vi "Sub_Read_Variable_Header.vi"(8 "error in (no error)":errorcluster, 9 "QoS":T1, 10 "Variable Header":u8[](array[numeric]) format="%x") -> (0 "error out":errorcluster, 1 "remaining bytes":u8[](array[numeric]) format="%x", 2 "Message ID":u16=1 format="%x", 3 "Topic Name":string="Topic")   [LabVIEW 2024, in "MQTT_Functions.lvlib"]
uses:
  MQTT_Functions.lvlib
  Controls/QoS.ctl
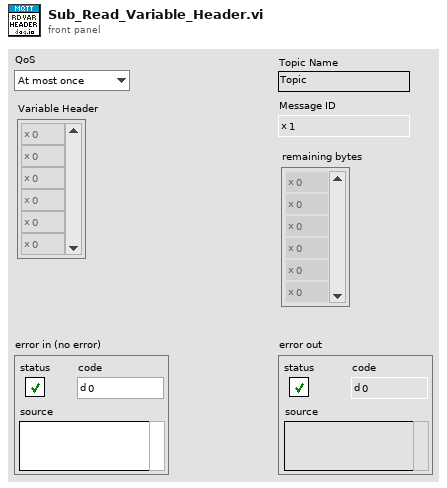
[diagram p1: front panel]
types:
  T1 = typedef "MQTT_Functions.lvlib/QoS.ctl" = enum8{"At most once", "At least once", "Exactly once", "Reserved"}
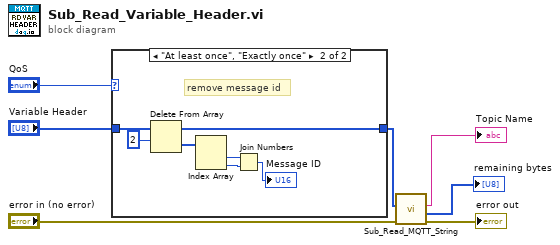
[diagram p0: block diagram]
diagram:
  n1 = case shown="\"At least once\", \"Exactly once\"" "QoS" {
    tunnel: "Variable Header" -> [w8 w15]
    tunnel: [w8 w9] -> w4
    frame "At most once", Default {
      # "no message id"
    }
    frame "At least once", "Exactly once" {
      # "remove message id"
      n2 = Delete From Array(array=w15, length=2) -> (deleted portion=w13:u8[], array with subset deleted=w9:u8[])  [unwired: 1 in]
      n3 = Index Array(array=w13) -> (element #1=w11:u8, element #2=w12:u8)  [unwired: 2 in]
      n4 = Join Numbers(hi=w11, lo=w12) -> ((hi.lo)=→"Message ID":u16)
    }
  }
  n5 = call "Sub_Read_MQTT_String.vi"("error in (no error)"="error in (no error)", "UTF8 Byte Array"=w4) -> ("error out"=→"error out":errorcluster, "remaining bytes"=→"remaining bytes":u8[], "String"=→"Topic Name":string)  [unwired: 7 in]
